vi "Start Scan (Relative [FLR]).vi"(7 "Micropulse # In":i32, 8 "error in (no error)":errorcluster, 9 "Inspection Type":T1 caption="Inspection Type [def: Conventional Tests]", 10 "Scan definition":T2 {"Inspection Resolution" format="%#_6f"; "Scan Length" format="%#_6f"}, 11 "Axis No.":u8=1) -> (0 "error out":errorcluster, 5 "Micropulse # Out":i32)   [LabVIEW 2026, in "MicroPulse_Driver.lvlib"]
uses:
  MicroPulse_Driver.lvlib
  Data/Datatypes/MP - fly scan range (relative).ctl
  Data/Datatypes/MP - inspection direction (relative).ctl
  Data/Datatypes/MP - fly inspection tests.ctl
  Data/Datatypes/MP - MSE Action Condition.ctl
  <instrlib>/Micropulse/Micropulse.lvlib
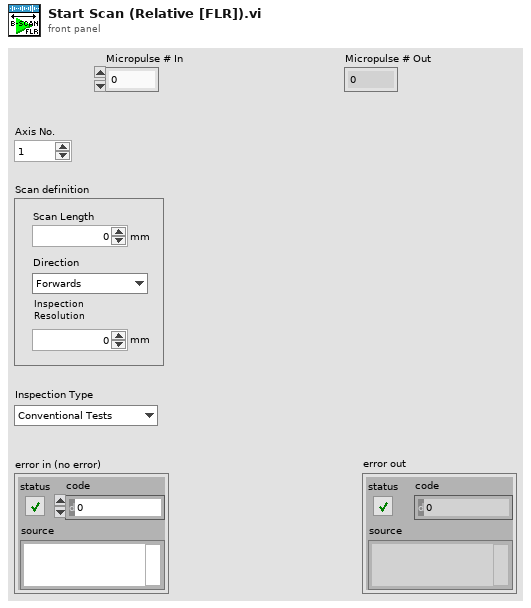
[diagram p1: front panel]
types:
  T1 = typedef "Micropulse.lvlib/MP - fly inspection tests.ctl" = enum16{"Conventional Tests", "Conv >> PA Tests", "PA >> Conv Tests", "PA Tests", "Group Tests", "PA Sweep as per FDEF"}
  T2 = typedef "Micropulse.lvlib/MP - fly scan range (relative).ctl" = cluster{"Scan Length":dbl, "Inspection Resolution":dbl, "Direction":T3}
  T3 = typedef "Micropulse.lvlib/MP - inspection direction (relative).ctl" = enum16{"Forwards", "Backwards", "Bidirectional"}
  T4 = typedef "Micropulse.lvlib/MP - MSE Action Condition.ctl" = enum16{"Normal Stop", "End of FLR or FLZ", "Stall", "Overshoot", "Any Axis Stop"}
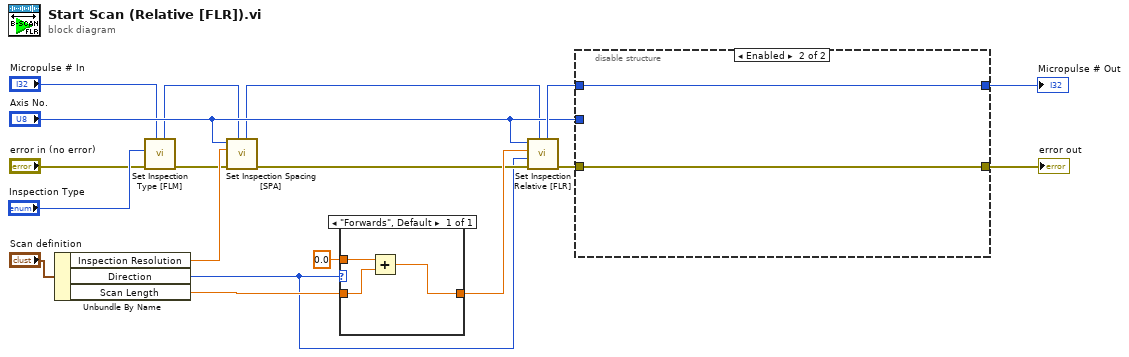
[diagram p0: block diagram]
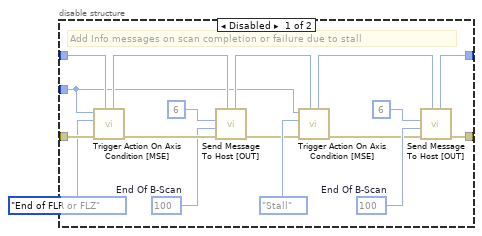
[diagram p2: hidden frame]
diagram:
  n1 = Unbundle By Name("Scan definition") -> ("Inspection Resolution"=w17:dbl, "Direction"=w6:T3, "Scan Length"=w16:dbl)
  n2 = call "Set Inspection Type [FLM].vi"("Micropulse # In"="Micropulse # In", "error in (no error)"="error in (no error)", "Inspection Type"="Inspection Type") -> ("error out"=w4:errorcluster, "Micropulse # Out"=w1:i32)  [unwired: 7 in]
  n3 = call "Set Inspection Spacing [SPA].vi"("Micropulse # In"=w1, "error in (no error)"=w4, "Spacing (mm)"=w17, "Axis No."="Axis No.") -> ("error out"=w8:errorcluster, "Micropulse # Out"=w9:i32)  [unwired: 6 in]
  n4 = case shown="\"Forwards\", Default" w6 {
    tunnel: w16 -> [w20]
    tunnel: [w19] -> w15
    tunnel: 0.0 ("Scan Start") -> [w21]
    frame "Forwards", Default {
      n5 = Add(x=w21, y=w20) -> (x+y=w19:dbl)
    }
  }
  n6 = call "Set Inspection Relative [FLR].vi"("Micropulse # In"=w9, "error in (no error)"=w8, "Direction"=w6, "End Location (mm)"=w15, "Axis No."="Axis No.") -> ("error out"=w14:errorcluster, "Micropulse # Out"=w13:i32)  [unwired: 5 in]
  n7 = disable-structure shown="Enabled" {
    disable-tunnel: w14 -> [w38 w39]
    disable-tunnel: w13 -> [w36 w40]
    disable-tunnel: [w25 w40] -> w12
    disable-tunnel: [w23 w39] -> w11
    disable-tunnel: "Axis No." -> [w22 _]
    frame Disabled {
      w31 = u8 100  # End Of B-Scan
      w32 = u8 100  # End Of B-Scan
      # "Add Info messages on scan completion or failure due to stall"
      n8 = call "Trigger Action On Axis Condition [MSE].vi"("Micropulse # In"=w36, "error in (no error)"=w38, "Action Condition"=MP_-_MSE_Action_Condition."End of FLR or FLZ", "Axis No."=w22) -> ("error out"=w35:errorcluster, "Micropulse # Out"=w34:i32)  [unwired: 6 in]
      n9 = call "Send Message To Host [OUT].vi"("Micropulse # In"=w34, "error in (no error)"=w35, "Parameter"=w32, "Header No."=u8 6) -> ("error out"=w24:errorcluster, "Micropulse # Out"=w26:i32)  [unwired: 6 in]
      n10 = call "Trigger Action On Axis Condition [MSE].vi"("Micropulse # In"=w26, "error in (no error)"=w24, "Action Condition"=MP_-_MSE_Action_Condition."Stall", "Axis No."=w22) -> ("error out"=w28:errorcluster, "Micropulse # Out"=w29:i32)  [unwired: 6 in]
      n11 = call "Send Message To Host [OUT].vi"("Micropulse # In"=w29, "error in (no error)"=w28, "Parameter"=w31, "Header No."=u8 6) -> ("error out"=w23:errorcluster, "Micropulse # Out"=w25:i32)  [unwired: 6 in]
    }
    frame Enabled {
    }
  }
  "error out" <- w11
  "Micropulse # Out" <- w12
